vi "ToRelativePath.vi"(11 "absolutely path":string) -> (3 "relative path":string)   [LabVIEW 2009]
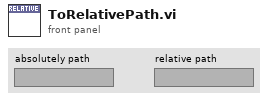
[diagram p1: front panel]
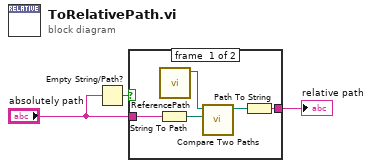
[diagram p0: block diagram]
diagram:
  n1 = Empty String/Path?(string/path="absolutely path") -> (empty?=w1:bool)
  n2 = case shown="True" w1 {
    tunnel: "absolutely path" -> [w8 w9]
    tunnel: [w6 w9] -> w3
    frame #0 {
      n3 = String To Path(string=w8) -> (path=w4:path)
      n4 = call "ReferencePath.vi"() -> ("relative path"=w5:path)  [unwired: 11 in]
      n5 = call <vilib>:"Compare Two Paths.vi"("Path 2"=w4, "Path 1"=w5) -> ("Relative Path from 1 to 2"=w7:path)  [unwired: 6 in, 3 out]
      n6 = Path To String(path=w7) -> (string=w6:string)
    }
    frame #1 {
    }
  }
  "relative path" <- w3
